vi "LHF.DB.Mongo.Util.FindEqual.vi"(8 "error in (no error)":errorcluster, 9 "Attribute":cluster{"name":string, "value":string}, 10 "Collection":string, 11 "LHF.DB.Mongo in":refnum<class "LHF.DB.Mongo.lvclass">) -> (0 "error out":errorcluster, 2 "Documents":string[](array[string]), 3 "LHF.DB.Mongo out":refnum<class "LHF.DB.Mongo.lvclass">, 5 "ObjectIDs":string[](array[string]))   [LabVIEW 2013, in "LHF.DB.Mongo.lvclass"]
uses:
  LHF.DB.Mongo.lvclass
  C:/Users/schim/Desktop/Projetos/LabVIEW-MongoDB/src/Driver/MongoDB.Bson.dll
  Driver/MongoDB.Bson.dll
  C:/Users/schim/Desktop/Projetos/LabVIEW-MongoDB/src/Driver/MongoDB.Driver.dll
  Driver/MongoDB.Driver.dll
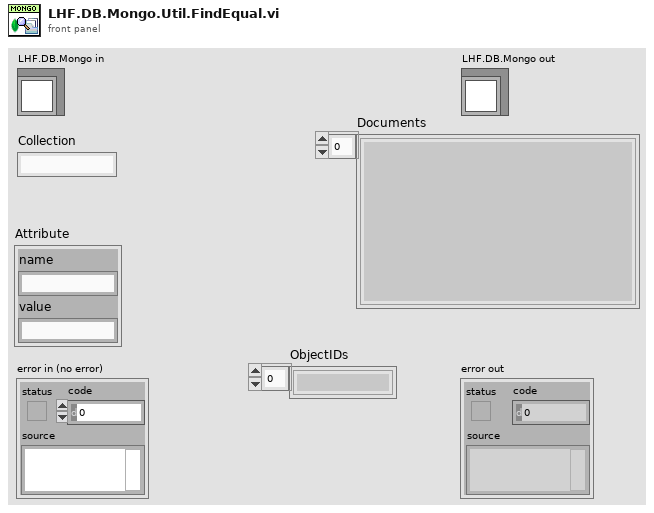
[diagram p1: front panel]
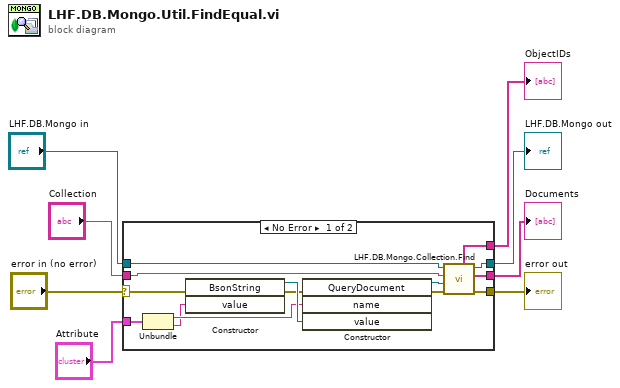
[diagram p0: block diagram]
diagram:
  n1 = case shown="No Error" "error in (no error)" {
    selector: "error in (no error)" -> [w17 w24]
    tunnel: [w12 w24] -> w7
    tunnel: [w10 w23] -> w5
    tunnel: "LHF.DB.Mongo in" -> [w16 w23]
    tunnel: "Collection" -> [w15 _]
    tunnel: "Attribute" -> [w21 _]
    tunnel: [w11 _] -> w2
    tunnel: [w9 _] -> w1
    frame No Error {
      n2 = Unbundle(w21) -> ("name"=w20:string, "value"=w19:string)
      n3 = constructor class="BsonString"(error in=w17, "value"=w19) -> (reference out=w22:refnum<k24>, error out=w18:errorcluster)  [unwired: 2 in, 2 out]
      n4 = constructor class="QueryDocument"(error in=w18, "name"=w20, "value"=w22) -> (reference out=w14:refnum<k24>, error out=w13:errorcluster)  [unwired: 2 in, 3 out]
      n5 = call "LHF.DB.Mongo.Collection.Find.vi"("error in (no error)"=w13, "query"=w14, "Collection"=w15, "LHF.DB.Mongo in"=w16) -> ("error out"=w12:errorcluster, "Documents"=w11:string[], "LHF.DB.Mongo out"=w10:refnum<class "LHF.DB.Mongo.lvclass">, "ObjectIDs"=w9:string[])  [unwired: 4 in]
    }
    frame Error {
    }
  }
  "error out" <- w7
  "LHF.DB.Mongo out" <- w5
  "Documents" <- w2
  "ObjectIDs" <- w1
